vi "Close MeasurementLink Session.vi"(8 "error in":errorcluster, 9 "initialize and close session behavior":T1, 10 "session in":variant, 11 "session factory in":refnum<class "Session Factory.lvclass">) -> (0 "error out":errorcluster)   [LabVIEW 2020, in "Plug-In SDK niDCPower Sessions.lvlib" / "Session Factory.lvclass"]
uses:
  Session Factory.lvclass
  <instrlib>/niDCPower/nidcpower.llb/niDCPower Close.vi
  <instrlib>/niDCPower/nidcpower.llb/niDCPower Detach gRPC session.vi
  Instrument Sessions/ISession Factory/ISession Factory.lvclass
  Instrument Sessions/ISession Factory/Initialize and Close Session Behavior.ctl
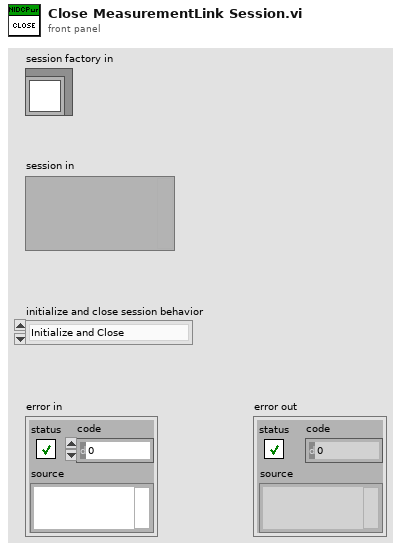
[diagram p1: front panel]
types:
  T1 = typedef "Plug-In SDK Instrument Sessions.lvlib/ISession Factory.lvclass/Initialize and Close Session Behavior.ctl" = enum16{"Initialize and Close", "Attach and Detach", "Initialize and Detach", "Attach and Close"}
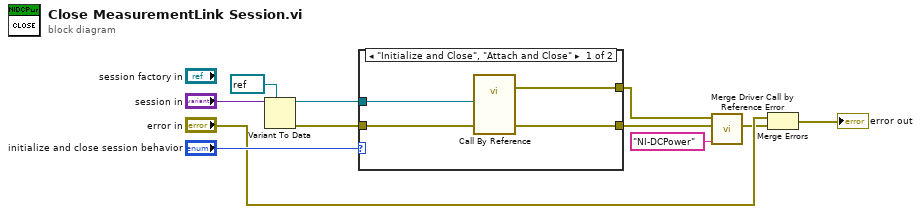
[diagram p0: block diagram]
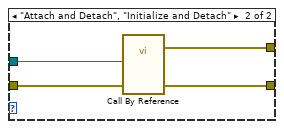
[diagram p2: hidden frame]
diagram:
  n1 = Variant To Data(type=refnum<k15> refnum ("instrument handle"), Variant="session in") -> (data=w7:refnum<k15>, error out=w8:errorcluster)  [unwired: 1 in]
  n2 = case shown="\"Initialize and Close\", \"Attach and Close\"" "initialize and close session behavior" {
    tunnel: w8 -> [w15 w19]
    tunnel: w7 -> [w14 w18]
    tunnel: [w13 w17] -> w2
    tunnel: [w12 w16] -> w3
    frame "Initialize and Close", "Attach and Close" {
      n3 = call-by-ref "?"("error in (no error)"=w15, "instrument handle"=w14) -> (error out=w12:errorcluster, 0:"error out"=w13:errorcluster)  [unwired: 11 in, 1 out]
    }
    frame "Attach and Detach", "Initialize and Detach" {
      n4 = call-by-ref "?"("error in (no error)"=w19, "instrument handle"=w18) -> (error out=w16:errorcluster, 0:"error out"=w17:errorcluster)  [unwired: 11 in, 1 out]
    }
  }
  n5 = call "Merge Driver Call by Reference Error.vi"("driver name"="NI-DCPower", "called vi error"=w2, "call by ref error"=w3) -> ("error out"=w1:errorcluster)  [unwired: 8 in]
  n6 = Merge Errors("error in", w1) -> (→"error out":errorcluster)
